vi "tool_Unicode_Convert ASCII to Unicode (2D).vi"(4 "ASCII":string[][](array[string])) -> (1 "Unicode":string[][](array[string]))   [LabVIEW 2009]
uses:
  kernel32.dll
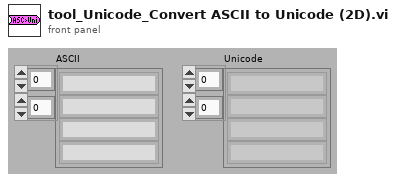
[diagram p1: front panel]
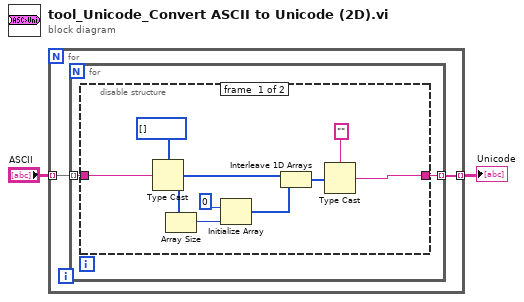
[diagram p0: block diagram]
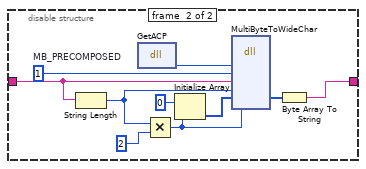
[diagram p2: hidden frame]
diagram:
  n1 = for {
    tunnel: "ASCII" -> [w4] mode=indexing
    tunnel: [w3] -> w1 mode=indexing
    n2 = for {
      tunnel: w4 -> [w6] mode=indexing
      tunnel: [w5] -> w3 mode=indexing
      n3 = disable-structure shown="Enabled" {
        disable-tunnel: w6 -> [w15 w18]
        disable-tunnel: [w7 w17] -> w5
        frame #0 {
          n4 = Type Cast(type=u8[] [], x=w15) -> (*(type *) &x=w11:u8[])
          n5 = Array Size(array=w11) -> (size(s)=w13:i32)
          n6 = Initialize Array(u8 0, w13) -> (w10:u8[])
          n7 = Interleave 1D Arrays(w11, w10) -> (w9:u8[])
          n8 = Type Cast(type="", x=w9) -> (*(type *) &x=w7:string)
        }
        frame #1 {
          w24 = u32 1  # MB_PRECOMPOSED
          n9 = String Length(string=w18) -> (length=w16:i32)
          n10 = dll-call lib="kernel32.dll" fn="GetACP" label="GetACP()"() -> (w19:u32)  [unwired: 3 in, 2 out]
          n11 = Multiply(x=w16, y=2) -> (x*y=w20:i32)
          n12 = Initialize Array(u8 0, w20) -> (w22:u8[])
          n13 = dll-call lib="kernel32.dll" fn="MultiByteToWideChar"("codePage"=w19, "dwFlags"=w24, "pMultiByteStr"=w18, "cbMultiByte"=w16, "lpWideCharStr"=w22, "cchWideChar"=w20) -> ("lpWideCharStr"=w21:u8[])  [unwired: 8 in, 3 out]
          n14 = Byte Array To String(unsigned byte array=w21) -> (string=w17:string)
        }
      }
    }
  }
  "Unicode" <- w1
